vi "path steer51.vi"(11 "lane":bool) -> (2 "curve vel limit":dbl=14.843332236967187, 3 "handle":dbl=-359.09688121459806)   [LabVIEW 2015]
uses:
  G_ALL.vi
  <vilib>/Analysis/polynomials.llb/1D Polynomial Evaluation (DBL).vi
  <vilib>/Analysis/polynomials.llb/nth Derivative of Polynomial (DBL).vi
  <vilib>/Analysis/polynomials.llb/Scalar Polynomial Evaluation (DBL).vi
  G_LCM.vi
  <vilib>/Analysis/NI_AALPro.lvlib
panel:
  in  "index (row)":i32
  out "Array 2":i32[](array[numeric])
  out "Polynomial Coefficients 3":dbl[][](array[numeric])
  out "Array":dbl[](array[numeric])
  out "dist speed":dbl[](array[numeric])=[-6.280629727990325, -5.767652620171672, -5.260811269352596, -4.750405616087261, -4.247626177640517, -3.7442417201726186, -3.234236998487254, -2.733202494381619, -2.2309876435732536, -1.727969770767316, -1.2170174151123292, -0.7112755506690004, -0.2048354308747279, 0.2980698513495696, 0.8052753145152414, 1.3068201262418702, 1.8071308154794987, 2.3105942059932456, 2.816881132611934, 3.321235349091914, 3.8262467144530254, 4.328309326210711, 4.83288013729348, 5.334580351902129, 5.8405154661100145, 6.344513436357381, 6.84671687285963, 7.347037647467956, 7.85260944831298, 8.355677730085302, 8.85924459600933, 9.36378646133383, 9.871392236798886, 10.379135157785838, 10.885149114578343, 11.386372469681485, 11.889282638845971, 12.390546046536894, 12.8945305329367, 13.394897794033318, 13.897303578434707, 14.398578387722258, 14.903133677335356, 15.408547950712162, 15.909840311837332, 16.412650077140604, 16.91886527417174, 17.42043178538479, 17.928892627599016, 18.429060187867897, 18.938769393907265, 19.44497971039645, 19.95108288625684, 20.458874628420645, 20.966711680341415, 21.468694651165553, 21.97077515459592, 22.476640025076534, 22.986901398368484, 23.490789085466282, 23.998423060461953, 24.50111144191703, 25.010444092843613]
  out "Polynomial Coefficients 2":dbl[](array[numeric])
  out "R0":dbl
  out "handle 2":dbl=-359.09688121459806
  out "dist":dbl[](array[numeric])=[-6.280629727990325, -5.767652620171672, -5.260811269352596, -4.750405616087261, -4.247626177640517, -3.7442417201726186, -3.234236998487254, -2.733202494381619, -2.2309876435732536, -1.727969770767316, -1.2170174151123292, -0.7112755506690004, -0.2048354308747279, 0.2980698513495696, 0.8052753145152414, 1.3068201262418702, 1.8071308154794987, 2.3105942059932456, 2.816881132611934, 3.321235349091914, 3.8262467144530254, 4.328309326210711, 4.83288013729348, 5.334580351902129, 5.8405154661100145, 6.344513436357381, 6.84671687285963, 7.347037647467956, 7.85260944831298, 8.355677730085302, 8.85924459600933, 9.36378646133383, 9.871392236798886, 10.379135157785838, 10.885149114578343, 11.386372469681485, 11.889282638845971, 12.390546046536894, 12.8945305329367, 13.394897794033318, 13.897303578434707, 14.398578387722258, 14.903133677335356, 15.408547950712162, 15.909840311837332, 16.412650077140604, 16.91886527417174, 17.42043178538479, 17.928892627599016, 18.429060187867897, 18.938769393907265, 19.44497971039645, 19.95108288625684, 20.458874628420645, 20.966711680341415, 21.468694651165553, 21.97077515459592, 22.476640025076534, 22.986901398368484, 23.490789085466282, 23.998423060461953, 24.50111144191703, 25.010444092843613]
  in  "ap[g]":dbl=0.01 format="%#_13g"
  in  "mu":dbl=0.005 format="%#_13g"
  in  "an[g]":dbl=-0.05 format="%#_13g"
  out "Waveform Graph 2":dynamicdata(graph)=[{"t0"=timestamp(3558070004.848593 s since 1904-01-01), "dt"=1.0, "Y"=[2.6999392249698047, 1.6951051020445074, 1.0707905056587288, 0.8180527212240709, 0.9190152508675626, 1.2963877361766827, 1.970624056488019, 3.4965104940836413, 201.6, 201.6, 201.6, 201.6, 201.6, 201.6, 201.6, 201.6, 201.6, 201.6, 201.6, 201.6, 201.6, 201.6, 201.6, 201.6, 201.6, 9.532169956190149, 6.2694973959061215, 4.816384979354145, 3.8625477434998605, 3.1463412301935363, 2.568397389060611, 2.09391085834571, 1.7118919309961866, 1.427834339946269, 1.2511128718613436, 1.190295122332855, 1.2494808598163556, 1.4335700986818793, 1.7728772048959551, 2.418642872855935, 5.241778140587992, 201.6, 201.6, 201.6, 201.6, 201.6, 201.6, 201.6, 201.6, 201.6, 201.6, 201.6, 201.6, 201.6, 201.6, 201.6, 201.6, 201.6, 201.6, 201.6, 201.6, 201.6, 201.6]}, {"t0"=timestamp(3558070004.848593 s since 1904-01-01), "dt"=1.0, "Y"=[2.6999392249698047, 1.6951051020445074, 1.0707905056587288, 0.8180527212240709, 0.9190152508675626, 1.2963877361766827, 1.970624056488019, 3.4965104940836413, 20.777549661712815, 20.247536270100138, 19.694565186792815, 19.13150029565853, 18.550539773696645, 17.955042408424784, 17.333744168195455, 16.696661871332914, 16.035950098109442, 15.342378965317303, 14.611756797060403, 13.845642849689991, 13.03348797188081, 12.172479477913956, 11.240920032490967, 10.230903985827208, 9.099530123436892, 7.81122506851608, 6.2694973959061215, 4.816384979354145, 3.8625477434998605, 3.1463412301935363, 2.568397389060611, 2.09391085834571, 1.7118919309961866, 1.427834339946269, 1.2511128718613436, 1.190295122332855, 1.2494808598163556, 1.4335700986818793, 1.7728772048959551, 2.418642872855935, 5.241778140587992, 201.6, 201.6, 201.6, 201.6, 201.6, 201.6, 201.6, 201.6, 201.6, 201.6, 201.6, 201.6, 201.6, 201.6, 201.6, 201.6, 201.6, 201.6, 201.6, 201.6, 201.6, 201.6]}, {"t0"=timestamp(0 s since 1904-01-01), "dt"=1.0, "Y"=[2.6999392249698047, 1.6951051020445074, 1.0707905056587288, 0.8180527212240709, 0.9190152508675626, 1.2963877361766827, 1.970624056488019, 3.4965104940836413, 7.108855050211476, 9.429067355168725, 11.308583683012714, 12.902067626338482, 14.32116957022803, 15.603166352532973, 16.797313219711075, 16.696661871332914, 16.035950098109442, 15.342378965317303, 14.611756797060403, 13.845642849689991, 13.03348797188081, 12.172479477913956, 11.240920032490967, 10.230903985827208, 9.099530123436892, 7.81122506851608, 6.2694973959061215, 4.816384979354145, 3.8625477434998605, 3.1463412301935363, 2.568397389060611, 2.09391085834571, 1.7118919309961866, 1.427834339946269, 1.2511128718613436, 1.190295122332855, 1.2494808598163556, 1.4335700986818793, 1.7728772048959551, 2.418642872855935, 5.241778140587992, 8.106464321213798, 10.208013173205686, 11.948130714804863, 13.453538277833673, 14.81058095698709, 16.061404030280418, 17.21131827924602, 18.303446987203408, 19.317614592377343, 20.299067875936583, 21.228923087902636, 22.11953935666036, 22.978461118838254, 23.806486212234905, 24.597587927766437, 25.364173907146245, 26.113789179785613, 26.848724907341754, 27.555251257689754, 28.249167970580274, 28.919921293974994, 29.58403363562809]}]
  out "map_track for speed":dbl[][](array[numeric])=[[-0.3545450857664302, -6.2388566107065655], [-0.27704582904833586, -5.731767488012998], [-0.20533240909466363, -5.230025183339917], [-0.13399376942622507, -4.724629566643976], [-0.06871872109144915, -4.226105412976658], [-0.005201324439524461, -3.7267443688985153], [0.05648658324735591, -3.2204841411632317], [0.11292137912439827, -2.7226380925511173], [0.1614318645585973, -2.2227716212056117], [0.20611921619876952, -1.7217426590032276], [0.2514800464586248, -1.2128077861289897], [0.2966935930855752, -0.7090910317401496], [0.3370616547081277, -0.204262333528494], [0.37465481783960886, 0.29723589874642653], [0.4044573002719885, 0.803565034690598], [0.43241637259429494, 1.3043299380582118], [0.4571121863051213, 1.8040307510959646], [0.45201550718714745, 2.307468343503967], [0.3863546760099802, 2.809479406443939], [0.25417130196906557, 3.2962038986449116], [0.06111432793630125, 3.7628573931364953], [-0.19013433422201217, 4.19753080604394], [-0.49758286654376527, 4.597614676463535], [-0.8530000954510649, 4.951707459126808], [-1.2554532803579177, 5.2583045461104865], [-1.6928943683564668, 5.508622840575976], [-2.155745510638023, 5.703500011438359], [-2.634513106918592, 5.848766890858279], [-3.129308121801891, 5.952597228699951], [-3.627772088541141, 6.020504297462557], [-4.130029041586696, 6.056802252968919], [-4.634539834160694, 6.06240172093335], [-5.142102959732917, 6.055821687131267], [-5.649843095559644, 6.057503437117642], [-6.155823778443234, 6.063306282752706], [-6.656719729677723, 6.081419751160103], [-7.158588084773581, 6.113773922489787], [-7.651740703683538, 6.203582042123632], [-8.131423336348554, 6.35819424879321], [-8.583409716824091, 6.572846776944994], [-9.005194999840848, 6.845809681440183], [-9.386776083797882, 7.170882459126112], [-9.72476913428849, 7.54549791275371], [-10.011412061388244, 7.961766359884512], [-10.239416063440592, 8.40820583660063], [-10.40783468222519, 8.881970365592638], [-10.516838106738941, 9.376310409640807], [-10.590206702194822, 9.872481765496081], [-10.62912705284488, 10.379450831978916], [-10.637432741269066, 10.879549426143232], [-10.61938203200132, 11.388938910345853], [-10.592347246602534, 11.894426798329851], [-10.558291863385081, 12.399382890965526], [-10.517428444424214, 12.90552776587841], [-10.478548864380736, 13.41187433647924], [-10.440437467355913, 13.912408475588894], [-10.405933723810719, 14.413302000807835], [-10.372241554466061, 14.918043622740504], [-10.343427469450347, 15.427490791324738], [-10.315674147163909, 15.930613593740642], [-10.290940898551378, 16.43764467659748], [-10.26753174415437, 16.939787704369788], [-10.243318891221465, 17.44854450978152]]
  out "Polynomial Coefficients":dbl[](array[numeric])=[0.3514314245197786, 0.08317550338697662, -0.0038021171840465, -0.00346461088477799, -0.0012982677212205788, -0.00011561582792426496]
  out "XY Graph":cluster{"Y":dbl[], "Y":dbl[]}[](graph)=[{"Y"=[-0.3545450857664302, -0.27704582904833586, -0.20533240909466363, -0.13399376942622507, -0.06871872109144915, -0.005201324439524461, 0.05648658324735591, 0.11292137912439827, 0.1614318645585973, 0.20611921619876952, 0.2514800464586248, 0.2966935930855752, 0.3370616547081277, 0.37465481783960886, 0.4044573002719885, 0.43241637259429494, 0.4571121863051213, 0.45201550718714745, 0.3863546760099802, 0.25417130196906557, 0.06111432793630125, -0.19013433422201217, -0.49758286654376527, -0.8530000954510649, -1.2554532803579177, -1.6928943683564668], "Y"=[-6.2388566107065655, -5.731767488012998, -5.230025183339917, -4.724629566643976, -4.226105412976658, -3.7267443688985153, -3.2204841411632317, -2.7226380925511173, -2.2227716212056117, -1.7217426590032276, -1.2128077861289897, -0.7090910317401496, -0.204262333528494, 0.29723589874642653, 0.803565034690598, 1.3043299380582118, 1.8040307510959646, 2.307468343503967, 2.809479406443939, 3.2962038986449116, 3.7628573931364953, 4.19753080604394, 4.597614676463535, 4.951707459126808, 5.2583045461104865, 5.508622840575976]}, {"Y"=[-0.34824861454222367, -0.2838190821086385, -0.21088307053199773, -0.13573975147394757, -0.06474548918773154, 0.0006618412479036939, 0.06025418227747581, 0.11267247761975072, 0.16039640436065217, 0.20497730506502992, 0.2486380781866307, 0.29146844512109193, 0.33431047405158726, 0.3757168715400785, 0.41343550897313974, 0.4415691081325965, 0.4528064519658091, 0.43617827243140883, 0.3771483424612058, 0.2619623140505302, 0.07848992524601944, -0.17634937336605716, -0.5008339909423127, -0.875287479505389, -1.27737354646982, -1.6668168609056053], "Y"=[-6.2388566107065655, -5.731767488012998, -5.230025183339917, -4.724629566643976, -4.226105412976658, -3.7267443688985153, -3.2204841411632317, -2.7226380925511173, -2.2227716212056117, -1.7217426590032276, -1.2128077861289897, -0.7090910317401496, -0.204262333528494, 0.29723589874642653, 0.803565034690598, 1.3043299380582118, 1.8040307510959646, 2.307468343503967, 2.809479406443939, 3.2962038986449116, 3.7628573931364953, 4.19753080604394, 4.597614676463535, 4.951707459126808, 5.2583045461104865, 5.508622840575976]}]
  out "ref":dbl[](array[numeric])=[-29.50710129286377, 0.08298448837840622, 0.3514314245197786]
  in  "gain":dbl[](array[numeric])=[0.7, 1400.0, 750.0]
  out "path end":bool
  out "map_track for steering":dbl[][](array[numeric])=[[-0.3545450857664302, -6.2388566107065655], [-0.27704582904833586, -5.731767488012998], [-0.20533240909466363, -5.230025183339917], [-0.13399376942622507, -4.724629566643976], [-0.06871872109144915, -4.226105412976658], [-0.005201324439524461, -3.7267443688985153], [0.05648658324735591, -3.2204841411632317], [0.11292137912439827, -2.7226380925511173], [0.1614318645585973, -2.2227716212056117], [0.20611921619876952, -1.7217426590032276], [0.2514800464586248, -1.2128077861289897], [0.2966935930855752, -0.7090910317401496], [0.3370616547081277, -0.204262333528494], [0.37465481783960886, 0.29723589874642653], [0.4044573002719885, 0.803565034690598], [0.43241637259429494, 1.3043299380582118], [0.4571121863051213, 1.8040307510959646], [0.45201550718714745, 2.307468343503967], [0.3863546760099802, 2.809479406443939], [0.25417130196906557, 3.2962038986449116], [0.06111432793630125, 3.7628573931364953], [-0.19013433422201217, 4.19753080604394], [-0.49758286654376527, 4.597614676463535], [-0.8530000954510649, 4.951707459126808], [-1.2554532803579177, 5.2583045461104865], [-1.6928943683564668, 5.508622840575976]]
  in  "control point":dbl=0.3 format="%#_13g"
  out "R_new":dbl=-132.87270287440214
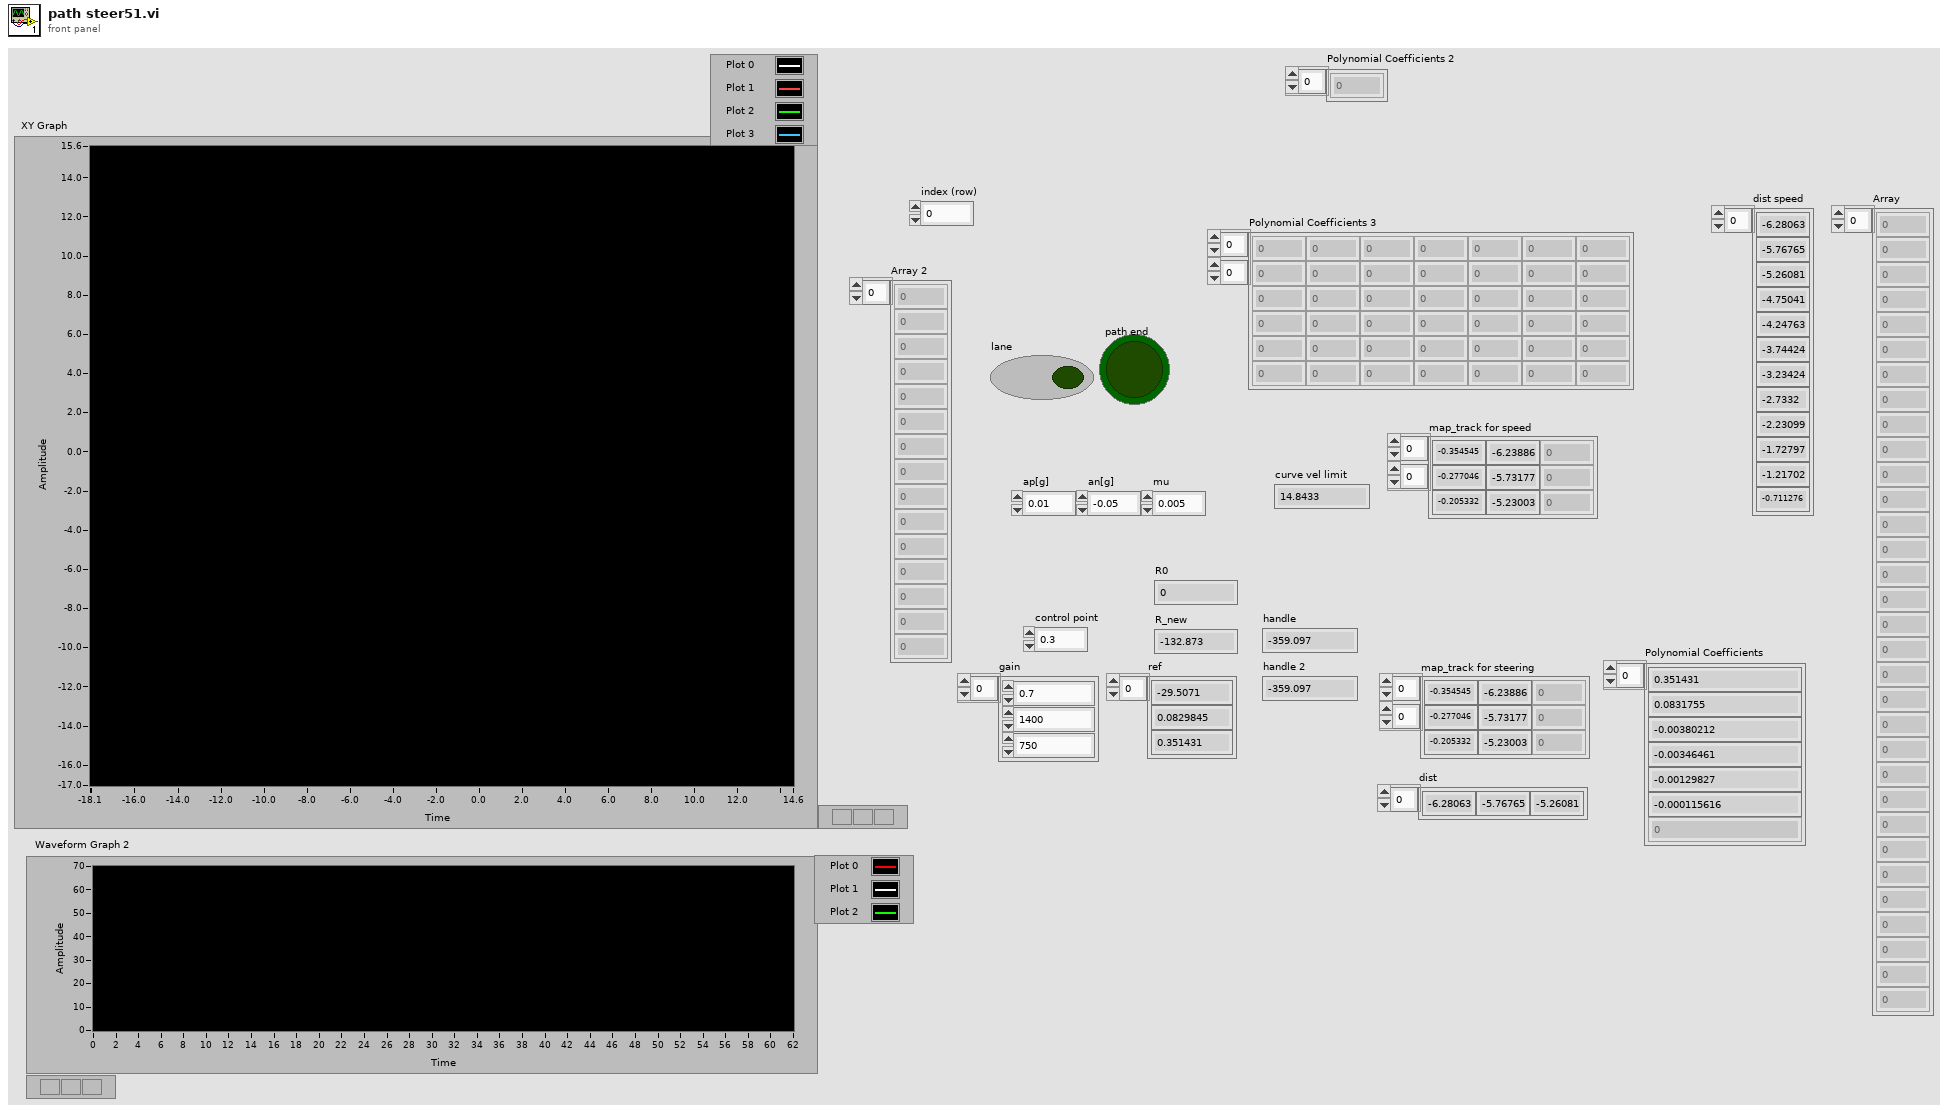
[diagram p1: front panel]
types:
  T1 = cluster{"Steer_input":dbl, "Steer_output":dbl, "VS_des":dbl, "VS_can":dbl, "heading":dbl, "auto":bool, "run":bool, "x":dbl, "y":dbl, "slam_y":dbl, "slam_x":dbl, "slam_heading":dbl}
  T2 = cluster{"C_Wheel base":dbl, "ratio_steer":dbl, "Overall width":dbl, "af":dbl, "turn radius":dbl, "eval":dbl, "ap":dbl, "an":dbl, "Vmax":dbl, "mu":dbl, "Vlast":dbl}
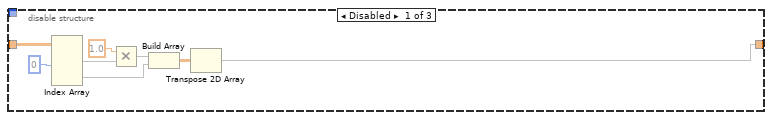
[diagram p2: hidden frame]
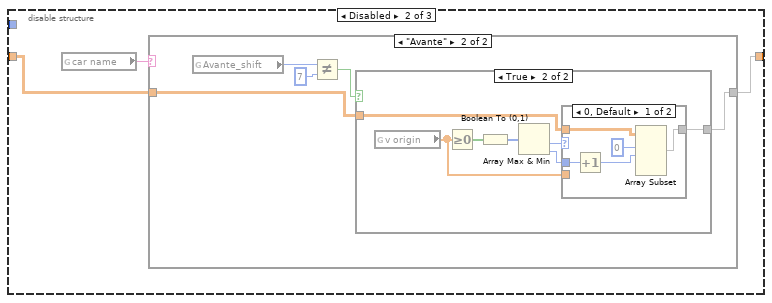
[diagram p3: hidden frame]
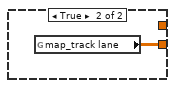
[diagram p7: hidden frame]
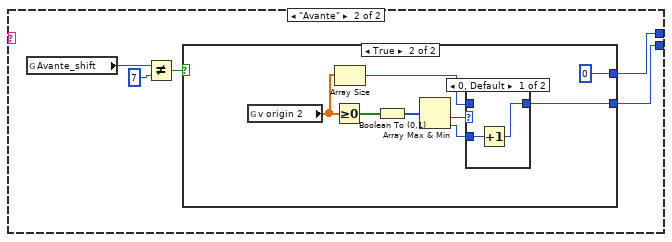
[diagram p9: hidden frame]
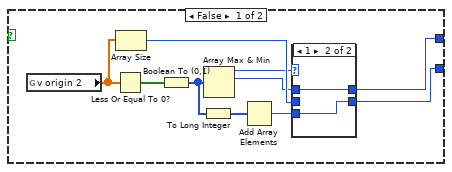
[diagram p10: hidden frame]
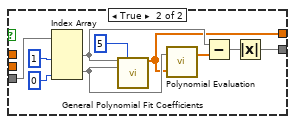
[diagram p14: hidden frame]
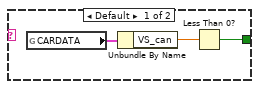
[diagram p17: hidden frame]
diagram:
  n1 = flat-sequence {
    tunnel: [w193] -> w1
    tunnel: w1 -> [w282]
    tunnel: [w357] -> w5
    tunnel: w5 -> [w373]
    tunnel: [w373] -> w4
    tunnel: [w364] -> w3
    tunnel: [w368] -> w2
    tunnel: w4 -> [w405]
    tunnel: w3 -> [w403]
    tunnel: w2 -> [w391]
    frame #0 {
      n2 = case shown="False" "lane" {
        tunnel: [w73 w116] -> w30
        tunnel: [w75 _] -> w64
        frame False {
          n3 = global read "G_ALL.vi" "current idx"() -> (w76:i32)
          n4 = Subtract(x=w76, y=2) -> (x-y=w83:i32)
          n5 = global read "G_ALL.vi" "map_track"() -> (w74:dbl[][])
          n6 = Max & Min(x=w83, y=0) -> (max(x,y)=w71:i32)  [unwired: 1 out]
          n7 = disable-structure shown="Enabled" {
            disable-tunnel: w74 -> [w92 w94 w115]
            disable-tunnel: [w85 w93 w115] -> w73
            disable-tunnel: w71 -> [_ _ _]
            frame Disabled {
              n8 = Index Array(array=w92, index (col) #1=0 ("disabled index (col)")) -> (element #1=w90:dbl[], element #2=w87:dbl[])  [unwired: 3 in]
              n9 = Multiply(x=1.0, y=w90) -> (x*y=w88:dbl[])
              n10 = Build Array(w88, w87) -> (w86:dbl[][])
              n11 = Transpose 2D Array(2D array=w86) -> (transposed array=w85:dbl[][])
            }
            frame Disabled {
              n12 = global read "G_LCM.vi" "car name"() -> (w95:string)
              n13 = case shown="\"Avante\"" w95 {
                tunnel: [w96 w98] -> w93
                tunnel: w94 -> [w96 w97]
                frame Default {
                }
                frame "Avante" {
                  n14 = global read "G_ALL.vi" "Avante_shift"() -> (w100:u8)
                  n15 = Not Equal?(x=w100, y=u8 7) -> (x != y?=w99:bool)
                  n16 = case shown="True" w99 {
                    tunnel: [_ w104] -> w98
                    tunnel: w97 -> [_ w103]
                    frame False {
                    }
                    frame True {
                      n17 = global read "G_ALL.vi" "v origin"() -> (w105:dbl[])
                      n18 = Greater Or Equal To 0?(x=w105) -> (x >= 0?=w108:bool[])
                      n19 = Boolean To (0,1)(Boolean=w108) -> (0, 1=w107:i16[])
                      n20 = Array Max & Min(array=w107) -> (min value=w106:i16, min index (indices)=w102:i32)  [unwired: 2 out]
                      n21 = case shown="0, Default" w106 {
                        tunnel: w105 -> [_ _]
                        tunnel: [w110 w114] -> w104
                        tunnel: w103 -> [w112 w114]
                        tunnel: w102 -> [w113 _]
                        frame 0, Default {
                          n22 = Increment(x=w113) -> (x+1=w111:i32)
                          n23 = Array Subset(array=w112, index (row)=0 ("index"), length (row)=w111) -> (w110:dbl[][])  [unwired: 2 in]
                        }
                        frame 1 {
                        }
                      }
                    }
                  }
                }
              }
            }
            frame Enabled {
            }
          }
          n24 = Array Subset(array=w73, index (row)=w71, length (row)=5 ("length")) -> (w80:dbl[][])  [unwired: 2 in]
          n25 = Index Array(array=w80, index (col)=1 ("disabled index (col)")) -> (element=w78:dbl[])  [unwired: 1 in]
          n26 = Threshold 1D Array(2:0.0 ("threshold y"), 3:w78) -> (0:w72:dbl)  [unwired: 1 in]
          n27 = Add(x=w71, y=w72) -> (x+y=w75:dbl)
        }
        frame True {
          n28 = global read "G_ALL.vi" "map_track lane"() -> (w116:dbl[][])
        }
      }
      n29 = Round Toward -Infinity(1:w64) -> (0:w59:dbl)
      n30 = Index Array(array=w30, index (col) #1=0 ("disabled index (col)")) -> (element #1=w22:dbl[], element #2=w23:dbl[])  [unwired: 3 in]
      n31 = Equal?(x=w59, y=w64) -> (x = y?=w60:bool)
      n32 = To Long Integer(number=w59) -> (32bit integer=w61:i32)
      n33 = Interpolate 1D Array(1:w64, 2:w22) -> (0:w24:dbl)
      n34 = Interpolate 1D Array(1:w64, 2:w23) -> (0:w25:dbl)
      n35 = Increment(x=w61) -> (x+1=w62:i32)
      n36 = Round Toward +Infinity(x=w64) -> (ceil(x): smallest int >= x=w58:dbl)
      n37 = Select(t=w61, s=w60, f=w62) -> (s? t:f=w18:i32)
      n38 = global read "G_ALL.vi" "CARDATA"() -> (w28:T1)
      n39 = Array Subset(array=w30, index (row)=0 ("index"), length (row)=w18) -> (w32:dbl[][])  [unwired: 2 in]
      n40 = Unbundle By Name(w28) -> ("VS_can"=w65:dbl)
      n41 = Index Array(array=w32, index (col) #1=0 ("disabled index (col)")) -> (element #1=w34:dbl[], element #2=w35:dbl[])  [unwired: 3 in]
      n42 = Reverse 1D Array(array=w34) -> (reversed array=w36:dbl[])
      n43 = Reverse 1D Array(array=w35) -> (reversed array=w37:dbl[])
      n44 = Multiply(x=2.0, y=w65) -> (x*y=w66:dbl)
      n45 = Build Array(w36, w37) -> (w56:dbl[][])
      n46 = To Long Integer(number=w58) -> (32bit integer=w9:i32)
      n47 = Max & Min(x=w66, y=25.0) -> (max(x,y)=w29:dbl)  [unwired: 1 out]
      n48 = Array Subset(array=w30, index (row)=w9) -> (w54:dbl[][])  [unwired: 3 in]
      n49 = Transpose 2D Array(2D array=w56) -> (transposed array=w57:dbl[][])
      n50 = Build Array(w24, w25) -> (w39:dbl[])
      n51 = for {
        tunnel: w57 -> [w119] mode=indexing
        shift-right: [w119] -> _
        shift-left: w39 -> [w126]
        shift-right: [w118] -> _
        shift-left: 0.0 -> [w121]
        tunnel: 15.0 ("y") -> [w120]
        tunnel: [w118] -> w43 mode=indexing
        stop <- w117 stop-if-true
        n52 = Subtract(x=w119, y=w126) -> (x-y=w125:dbl[])
        n53 = Square(x=w125) -> (x^2=w124:dbl[])
        n54 = Add Array Elements(numeric array=w124) -> (sum=w123:dbl)
        n55 = Square Root(x=w123) -> (sqrt(x)=w122:dbl)
        n56 = Add(x=w121, y=w122) -> (x+y=w118:dbl)
        n57 = Greater Or Equal?(x=w118, y=w120) -> (x >= y?=w117:bool)
      }
      n58 = for {
        tunnel: w54 -> [w129] mode=indexing
        shift-right: [w129] -> _
        shift-left: w39 -> [w136]
        shift-right: [w128] -> _
        shift-left: 0.0 -> [w131]
        tunnel: w29 -> [w130]
        tunnel: [w128] -> w55 mode=indexing
        tunnel: [w127] -> w69
        stop <- w127 stop-if-true
        n59 = Subtract(x=w129, y=w136) -> (x-y=w135:dbl[])
        n60 = Square(x=w135) -> (x^2=w134:dbl[])
        n61 = Add Array Elements(numeric array=w134) -> (sum=w133:dbl)
        n62 = Square Root(x=w133) -> (sqrt(x)=w132:dbl)
        n63 = Add(x=w131, y=w132) -> (x+y=w128:dbl)
        n64 = Greater Or Equal?(x=w128, y=w130) -> (x >= y?=w127:bool)
      }
      n65 = global read "G_ALL.vi" "v origin"() -> (w10:dbl[])
      n66 = Array Subset(array=w10, index=0, length=w18) -> (w16:dbl[])
      n67 = Negate(x=w43) -> (-x=w41:dbl[])
      n68 = Not(x=w69) -> (.not. x?=→"path end":bool)
      n69 = Array Size(array=w43) -> (size(s)=w13:i32)
      n70 = Array Size(array=w55) -> (size(s)=w8:i32)
      n71 = Reverse 1D Array(array=w16) -> (reversed array=w15:dbl[])
      n72 = Array Subset(array=w10, index=w9, length=w8) -> (w7:dbl[])
      n73 = Reverse 1D Array(array=w41) -> (reversed array=w42:dbl[])
      n74 = Array Subset(array=w57, index (row)=0 ("index"), length (row)=w13) -> (w49:dbl[][])  [unwired: 2 in]
      n75 = Array Subset(array=w54, index (row)=0 ("index"), length (row)=w8) -> (w68:dbl[][])  [unwired: 2 in]
      n76 = Build Array (concatenate)(w42, w55) -> (w19:dbl[])
      n77 = Array Subset(array=w15, index=0, length=w13) -> (w12:dbl[])
      n78 = global write "G_ALL.vi" "dist"(w19) -> ()
      n79 = Reverse 1D Array(array=w12) -> (reversed array=w11:dbl[])
      n80 = Index Array(array=w49, index (col) #1=0 ("disabled index (col)")) -> (element #1=w50:dbl[], element #2=w51:dbl[])  [unwired: 3 in]
      n81 = Reverse 1D Array(array=w50) -> (reversed array=w47:dbl[])
      n82 = Reverse 1D Array(array=w51) -> (reversed array=w46:dbl[])
      n83 = Build Array (concatenate)(w11, w7) -> (w6:dbl[])
      n84 = Build Array(w47, w46) -> (w45:dbl[][])
      n85 = global write "G_ALL.vi" "v origin 2"(w6) -> ()
      n86 = Transpose 2D Array(2D array=w45) -> (transposed array=w52:dbl[][])
      n87 = Build Array (concatenate)(w52, w68) -> (w20:dbl[][])
      n88 = global write "G_ALL.vi" "map_track 2"(w20) -> ()
    }
    frame #1 {
      n89 = disable-structure shown="Disabled" {
        disable-tunnel: [w157 _] -> w145
        frame Disabled {
          n90 = global read "G_LCM.vi" "car name"() -> (w157:string)
        }
        frame Enabled {
        }
      }
      n91 = case shown="\"False\", Default" w145 {
        tunnel: [w158 w162] -> w141
        tunnel: [_ w161] -> w140
        frame "False", Default {
          n92 = global read "G_ALL.vi" "dist"() -> (w159:dbl[])
          n93 = Array Size(array=w159) -> (size(s)=w158:i32)
        }
        frame "Avante" {
          n94 = global read "G_ALL.vi" "Avante_shift"() -> (w163:u8)
          n95 = Not Equal?(x=w163, y=u8 7) -> (x != y?=w160:bool)
          n96 = case shown="True" w160 {
            tunnel: [w168 w183] -> w162
            tunnel: [w172 0] -> w161
            frame False {
              n97 = global read "G_ALL.vi" "v origin 2"() -> (w174:dbl[])
              n98 = Less Or Equal To 0?(x=w174) -> (x <= 0?=w169:bool[])
              n99 = Array Size(array=w174) -> (size(s)=w173:i32)
              n100 = Boolean To (0,1)(Boolean=w169) -> (0, 1=w166:i16[])
              n101 = To Long Integer(number=w166) -> (32bit integer=w165:i32[])
              n102 = Array Max & Min(array=w166) -> (max value=w170:i16, max index (indices)=w171:i32)  [unwired: 2 out]
              n103 = Add Array Elements(numeric array=w165) -> (sum=w167:i32)
              n104 = case shown="1" w170 {
                tunnel: w173 -> [w175 _]
                tunnel: [_ w177] -> w172
                tunnel: w171 -> [_ w177]
                tunnel: [w175 w176] -> w168
                tunnel: w167 -> [_ w176]
                frame 0, Default {
                }
                frame 1 {
                }
              }
            }
            frame True {
              n105 = global read "G_ALL.vi" "v origin 2"() -> (w180:dbl[])
              n106 = Greater Or Equal To 0?(x=w180) -> (x >= 0?=w185:bool[])
              n107 = Array Size(array=w180) -> (size(s)=w184:i32)
              n108 = Boolean To (0,1)(Boolean=w185) -> (0, 1=w182:i16[])
              n109 = Array Max & Min(array=w182) -> (min value=w181:i16, min index (indices)=w178:i32)  [unwired: 2 out]
              n110 = case shown="0, Default" w181 {
                tunnel: w184 -> [_ w188]
                tunnel: [w187 w188] -> w183
                tunnel: w178 -> [w186 _]
                frame 0, Default {
                  n111 = Increment(x=w186) -> (x+1=w187:i32)
                }
                frame 1 {
                }
              }
            }
          }
        }
      }
      n112 = global read "G_ALL.vi" "dist"() -> (w144:dbl[])
      n113 = Array Subset(array=w144, index=w140, length=w141) -> (w137:dbl[])
      "dist speed" <- w137
      n114 = Threshold 1D Array(2:-6.0 ("threshold y"), 3:w137) -> (0:w155:dbl)  [unwired: 1 in]
      n115 = Round Toward -Infinity(1:w155) -> (0:w156:dbl)
      n116 = To Long Integer(number=w156) -> (32bit integer=w147:i32)
      n117 = Array Subset(array=w137, index=w147) -> (→"dist":dbl[])  [unwired: 1 in]
      n118 = Threshold 1D Array(1:w147, 2:6.0 ("threshold y"), 3:w137) -> (0:w150:dbl)
      n119 = Round Toward +Infinity(x=w150) -> (ceil(x): smallest int >= x=w149:dbl)
      n120 = global read "G_ALL.vi" "map_track 2"() -> (w143:dbl[][])
      n121 = To Long Integer(number=w149) -> (32bit integer=w151:i32)
      n122 = Subtract(x=w151, y=w147) -> (x-y=w152:i32)
      n123 = Increment(x=w152) -> (x+1=w153:i32)
      n124 = Array Subset(array=w143, index (row)=w140) -> (w142:dbl[][])  [unwired: 3 in]
      n125 = Array Subset(array=w142, index (row)=w147) -> (→"map_track for speed":dbl[][])  [unwired: 3 in]
      n126 = Array Subset(array=w142, index (row)=w147, length (row)=w153) -> (→"map_track for steering":dbl[][])  [unwired: 2 in]
    }
    frame #2 {
      n127 = local read "dist speed"() -> (w198:dbl[])
      n128 = local read "map_track for speed"() -> (w199:dbl[][])
      n129 = Multiply(x=w198, y=0.0) -> (x*y=w196:dbl[])
      n130 = Add(x=w196, y=inf) -> (x+y=w194:dbl[])
      n131 = while {
        shift-right: [w210] -> _
        shift-left: w199 -> [w217]
        tunnel: w198 -> [w214]
        shift-right: [w211] -> w193
        shift-left: w194 -> [w213]
        tunnel: [w212] -> w192 mode=indexing
        tunnel: [w200] -> w189 mode=indexing
        stop <- w204 stop-if-true
        n132 = Array Size(array=w217) -> (size(s)=w219:i32[])
        n133 = Index Array(array=w219, index=0) -> (element=w215:i32)
        n134 = while {
          tunnel: w217 -> [w254]
          shift-right: [w252] -> _
          shift-left: w215 -> [w248]
          tunnel: [w248] -> w200
          tunnel: [w241] -> w212
          stop <- w250 stop-if-true
          n135 = disable-structure shown="Enabled" {
            disable-tunnel: w254 -> [w275 w277]
            disable-tunnel: [w274 w277] -> w247
            disable-tunnel: w248 -> [w273 _]
            frame Enabled {
              n136 = Array Subset(array=w275, index (row)=0 ("index"), length (row)=w273) -> (w274:dbl[][])  [unwired: 2 in]
            }
            frame Disabled {
            }
          }
          n137 = Scale By Power Of 2(n=i16 -1, x=w248) -> (x*2^n=w252:i32)
          n138 = Index Array(array=w247, index (col) #1=0 ("disabled index (col)")) -> (element #1=w258:dbl[], element #2=w256:dbl[])  [unwired: 3 in]
          n139 = call <vilib>:"General Polynomial Fit Coefficients.vi"("Y"=w258, "polynomial order"=5, "X"=w256) -> ("Polynomial Coefficients"=w240:dbl[])  [unwired: 11 in, 1 out]
          n140 = call-poly <vilib>:"Polynomial Evaluation.vi"("P(x)"=w240, "A"=w256) -> ("P(A)"=w255:dbl[])  [unwired: 1 out]
          n141 = Index Array(array=w240, index=5) -> (element=w239:dbl)
          n142 = Absolute Value(x=w239) -> (abs(x)=w238:dbl)
          n143 = Subtract(x=w258, y=w255) -> (x-y=w257:dbl[])
          n144 = Absolute Value(x=w257) -> (abs(x)=w242:dbl[])
          n145 = Greater Or Equal?(x=w238, y=1.0) -> (x >= y?=w244:bool)
          n146 = case shown="False" w244 {
            tunnel: w247 -> [_ w266]
            tunnel: [w262 w264] -> w243
            tunnel: w242 -> [w262 _]
            tunnel: [w261 w263] -> w241
            tunnel: w240 -> [w261 _]
            frame False {
            }
            frame True {
              n147 = Index Array(array=w266, index (col) #1=1 ("disabled index (col)"), index (col) #2=0 ("index (col)")) -> (element #1=w269:dbl[], element #2=w271:dbl[])  [unwired: 2 in]
              n148 = call <vilib>:"General Polynomial Fit Coefficients.vi"("Y"=w269, "polynomial order"=5, "X"=w271) -> ("Polynomial Coefficients"=w263:dbl[])  [unwired: 11 in, 1 out]
              n149 = call-poly <vilib>:"Polynomial Evaluation.vi"("P(x)"=w263, "A"=w271) -> ("P(A)"=w272:dbl[])  [unwired: 1 out]
              n150 = Subtract(x=w269, y=w272) -> (x-y=w270:dbl[])
              n151 = Absolute Value(x=w270) -> (abs(x)=w264:dbl[])
            }
          }
          n152 = Array Max & Min(array=w243) -> (max value=w251:dbl)  [unwired: 3 out]
          n153 = Less?(x=w251, y=0.05) -> (x < y?=w250:bool)
        }
        n154 = Less Or Equal?(x=w200, y=5) -> (x <= y?=w201:bool)
        n155 = Delete From Array(array=w217, length=w200, index (row)=0) -> (array with subset deleted=w210:dbl[][])  [unwired: 1 in, 1 out]
        n156 = Empty Array?(array=w210) -> (empty?=w206:bool)
        n157 = case shown="False" w201 {
          tunnel: w214 -> [w225 _]
          tunnel: w213 -> [w223 w237]
          tunnel: w212 -> [w221 _]
          tunnel: [w220 w237] -> w211
          frame False {
            n158 = call-poly <vilib>:"nth Derivative of Polynomial.vi"("order"=2, "P(x)"=w221) -> ("Nth Derivative of P(x)"=w228:dbl[])  [unwired: 8 in, 1 out]
            n159 = call-poly <vilib>:"nth Derivative of Polynomial.vi"("order"=1, "P(x)"=w221) -> ("Nth Derivative of P(x)"=w230:dbl[])  [unwired: 8 in, 1 out]
            n160 = call-poly <vilib>:"Polynomial Evaluation.vi"("P(x)"=w228, "A"=w225) -> ("P(A)"=w226:dbl[])  [unwired: 1 out]
            n161 = call-poly <vilib>:"Polynomial Evaluation.vi"("P(x)"=w230, "A"=w225) -> ("P(A)"=w234:dbl[])  [unwired: 1 out]
            n162 = Square(x=w234) -> (x^2=w231:dbl[])
            n163 = Increment(x=w231) -> (x+1=w233:dbl[])
            n164 = Square Root(x=w233) -> (sqrt(x)=w232:dbl[])
            n165 = Multiply(x=w232, y=w233) -> (x*y=w229:dbl[])
            n166 = Divide(x=w226, y=w229) -> (x/y=w236:dbl[])
            n167 = Reciprocal(x=w236) -> (1/x=w224:dbl[])
            n168 = Absolute Value(x=w224) -> (abs(x)=w222:dbl[])
            n169 = Max & Min(x=w222, y=w223) -> (min(x,y)=w220:dbl[])  [unwired: 1 out]
          }
          frame True {
          }
        }
        n170 = Array Size(array=w210) -> (size(s)=w209:i32[])
        n171 = Index Array(array=w209, index=0) -> (element=w203:i32)
        n172 = Less Or Equal?(x=w203, y=5) -> (x <= y?=w205:bool)
        n173 = Compound Arithmetic op=OR(w206, w205) -> (w204:bool)
      }
      "Array" <- w193
      "Polynomial Coefficients 3" <- w192
      "Array 2" <- w189
      n174 = Index Array(array=w192, index (row)="index (row)") -> (element=→"Polynomial Coefficients 2":dbl[])  [unwired: 1 in]
    }
    frame #3 {
      n175 = Compound Arithmetic op=MULTIPLY(w282, 9.81 ("value"), "mu") -> (w305:dbl[])
      n176 = Square Root(x=w305) -> (sqrt(x)=w280:dbl[])
      n177 = In Range and Coerce(upper limit=56.0 ("value"), x=w280, lower limit=0.5) -> (coerced(x)=w281:dbl[])  [unwired: 1 out]
      n178 = local read "path end"() -> (w312:bool)
      n179 = call "Convert to Dynamic Data6"("Array"=w281) -> ("Dynamic Data Type"=w287:dynamicdata)  [unwired: 3 in]
      n180 = Reverse 1D Array(array=w281) -> (reversed array=w313:dbl[])
      n181 = case shown="True" w312 {
        tunnel: w313 -> [w333 w337]
        tunnel: [w333 w336] -> w314
        frame False {
        }
        frame True {
          n182 = Replace Array Subset(array=w337, new element=0.0 ("new element/subarray"), index=0) -> (w336:dbl[])
        }
      }
      n183 = local read "dist speed"() -> (w285:dbl[])
      n184 = Array Size(array=w314) -> (size(s)=w310:i32)
      n185 = Reverse 1D Array(array=w285) -> (reversed array=w307:dbl[])
      n186 = Decrement(x=w310) -> (x-1=w309:i32)
      n187 = Negate(x=w307) -> (-x=w308:dbl[])
      n188 = for {
        N: w309 -> [_]
        tunnel: w314 -> [w353] mode=indexing
        tunnel: w308 -> [w354]
        shift-right: [w344] -> w293
        shift-left: w314 -> [w347]
        tunnel: w308 -> [w341] mode=indexing
        tunnel: "an[g]" -> [w338]
        i -> [w355]
        n189 = Square(x=w353) -> (x^2=w352:dbl)
        n190 = Increment(x=w355) -> (x+1=w346:i32)
        n191 = Array Subset(array=w347, index=w346) -> (w348:dbl[])  [unwired: 1 in]
        n192 = Array Subset(array=w354, index=w346) -> (w342:dbl[])  [unwired: 1 in]
        n193 = Subtract(x=w342, y=w341) -> (x-y=w340:dbl[])
        n194 = Compound Arithmetic op=MULTIPLY(w340, 9.81 ("value"), 2.0 ("value"), w338) -> (w350:dbl[])
        n195 = Subtract(x=w352, y=w350) -> (x-y=w349:dbl[])
        n196 = Square Root(x=w349) -> (sqrt(x)=w343:dbl[])
        n197 = Max & Min(x=w348, y=w343) -> (min(x,y)=w345:dbl[])  [unwired: 1 out]
        n198 = Replace Array Subset(array=w347, new element=w345, index=w346) -> (w344:dbl[])
      }
      n199 = Reverse 1D Array(array=w293) -> (reversed array=w290:dbl[])
      n200 = local read "dist speed"() -> (w284:dbl[])
      n201 = Array Size(array=w290) -> (size(s)=w296:i32)
      n202 = call "Convert to Dynamic Data5"("Array"=w290) -> ("Dynamic Data Type"=w286:dynamicdata)  [unwired: 3 in]
      n203 = Decrement(x=w296) -> (x-1=w297:i32)
      n204 = Negate(x=w284) -> (-x=w292:dbl[])
      n205 = for {
        N: w297 -> [_]
        tunnel: w290 -> [w330] mode=indexing
        tunnel: w292 -> [w331]
        shift-right: [w321] -> w289
        shift-left: w290 -> [w324]
        tunnel: w292 -> [w318] mode=indexing
        tunnel: "ap[g]" -> [w315]
        i -> [w332]
        n206 = Square(x=w330) -> (x^2=w329:dbl)
        n207 = Increment(x=w332) -> (x+1=w323:i32)
        n208 = Array Subset(array=w324, index=w323) -> (w325:dbl[])  [unwired: 1 in]
        n209 = Array Subset(array=w331, index=w323) -> (w319:dbl[])  [unwired: 1 in]
        n210 = Subtract(x=w319, y=w318) -> (x-y=w317:dbl[])
        n211 = Compound Arithmetic op=MULTIPLY(w317, 9.81 ("value"), 2.0 ("value"), w315) -> (w327:dbl[])
        n212 = Subtract(x=w329, y=w327) -> (x-y=w326:dbl[])
        n213 = Square Root(x=w326) -> (sqrt(x)=w320:dbl[])
        n214 = Max & Min(x=w325, y=w320) -> (min(x,y)=w322:dbl[])  [unwired: 1 out]
        n215 = Replace Array Subset(array=w324, new element=w322, index=w323) -> (w321:dbl[])
      }
      n216 = local read "dist speed"() -> (w283:dbl[])
      n217 = Threshold 1D Array(2:0.0 ("threshold y"), 3:w283) -> (0:w301:dbl)  [unwired: 1 in]
      n218 = call "Convert to Dynamic Data7"("Array"=w289) -> ("Dynamic Data Type"=w294:dynamicdata)  [unwired: 3 in]
      n219 = Interpolate 1D Array(1:w301, 2:w289) -> (0:w288:dbl)
      n220 = Merge Signals(w287, w286, w294) -> (w299:dynamicdata)
      n221 = Multiply(x=w288, y=3.6) -> (x*y=→"curve vel limit":dbl)
      n222 = Multiply(x=w299, y=3.6) -> (x*y=→"Waveform Graph 2":dynamicdata)
    }
    frame #4 {
      n223 = local read "map_track for steering"() -> (w363:dbl[][])
      n224 = Index Array(array=w363, index (col) #1=0 ("disabled index (col)")) -> (element #1=w360:dbl[], element #2=w361:dbl[])  [unwired: 3 in]
      n225 = call <vilib>:"General Polynomial Fit Coefficients.vi"("Y"=w360, "polynomial order"=5, "X"=w361) -> ("Polynomial Coefficients"=w356:dbl[])  [unwired: 11 in, 1 out]
      "Polynomial Coefficients" <- w356
      n226 = call-poly <vilib>:"Polynomial Evaluation.vi"("P(x)"=w356, "a"=0.0) -> ("P(a)"=w357:dbl)  [unwired: 1 out]
    }
    frame #5 {
      n227 = global read "G_LCM.vi" "car name"() -> (w369:string)
      n228 = case shown="\"Avante\"" w369 {
        tunnel: [w374 w377] -> w368
        frame Default {
          n229 = global read "G_ALL.vi" "CARDATA"() -> (w376:T1)
          n230 = Unbundle By Name(w376) -> ("VS_can"=w375:dbl)
          n231 = Less Than 0?(x=w375) -> (x < 0?=w374:bool)
        }
        frame "Avante" {
          n232 = global read "G_ALL.vi" "Avante_shift"() -> (w379:u8)
          n233 = Equal?(x=w379, y=u8 7) -> (x = y?=w377:bool)
        }
      }
      n234 = local read "Polynomial Coefficients"() -> (w372:dbl[])
      n235 = Negate(x="control point") -> (-x=w367:dbl)
      n236 = Select(t=w367, s=w368, f="control point") -> (s? t:f=w365:dbl)
      n237 = call-poly <vilib>:"nth Derivative of Polynomial.vi"("order"=1, "P(x)"=w372) -> ("Nth Derivative of P(x)"=w370:dbl[])  [unwired: 8 in, 1 out]
      n238 = call-poly <vilib>:"Polynomial Evaluation.vi"("P(x)"=w370, "a"=w365) -> ("P(a)"=w364:dbl)  [unwired: 1 out]
    }
    frame #6 {
      n239 = Square(x=w403) -> (x^2=w432:dbl)
      n240 = global read "G_ALL.vi" "CARDATA"() -> (w402:T1)
      n241 = Increment(x=w432) -> (x+1=w430:dbl)
      n242 = local read "Polynomial Coefficients"() -> (w404:dbl[])
      n243 = local read "Polynomial Coefficients"() -> (w385:dbl[])
      n244 = Unbundle By Name(w402) -> ("VS_can"=w401:dbl)
      n245 = Square Root(x=w430) -> (sqrt(x)=w431:dbl)
      n246 = Multiply(x=w431, y=w430) -> (x*y=w429:dbl)
      n247 = local read "control point"() -> (w382:dbl)
      n248 = Divide(x=w401, y=3.6) -> (x/y=w422:dbl)
      n249 = Absolute Value(x=w422) -> (abs(x)=w425:dbl)
      n250 = call-poly <vilib>:"nth Derivative of Polynomial.vi"("order"=2, "P(x)"=w404) -> ("Nth Derivative of P(x)"=w380:dbl[])  [unwired: 8 in, 1 out]
      n251 = Index Array(array=w385, index=1) -> (element=w383:dbl)
      n252 = call-poly <vilib>:"Polynomial Evaluation.vi"("P(x)"=w380, "a"=w382) -> ("P(a)"=w381:dbl)  [unwired: 1 out]
      n253 = Square(x=w383) -> (x^2=w388:dbl)
      n254 = Inverse Tangent(1:w383) -> (0:w427:dbl)
      n255 = Max & Min(x=w425, y=1.0) -> (max(x,y)=w423:dbl)  [unwired: 1 out]
      n256 = global read "G_ALL.vi" "CARSPEC"() -> (w417:T2)
      n257 = Divide(x=w405, y=w423) -> (x/y=w406:dbl)
      n258 = Divide(x=w429, y=w381) -> (x/y=w409:dbl)
      "R_new" <- w409
      n259 = Increment(x=w388) -> (x+1=w390:dbl)
      n260 = call "headingoperater.vi"("h1"=w427, "h2"=3.141592653589793) -> ("h2-h1"=w428:dbl)  [unwired: 8 in, 1 out]
      n261 = Unbundle By Name(w417) -> ("ratio_steer"=w419:dbl, "C_Wheel base"=w418:dbl)
      n262 = Select(t=w428, s=w391, f=w427) -> (s? t:f=w407:dbl)
      n263 = Square Root(x=w390) -> (sqrt(x)=w389:dbl)
      n264 = Multiply(x=w389, y=w390) -> (x*y=w387:dbl)
      n265 = Divide(x=w418, y=w409) -> (x/y=w411:dbl)
      n266 = Divide(x=w387, y=w381) -> (x/y=→"R0":dbl)
      n267 = Inverse Tangent(1:w411) -> (0:w413:dbl)
      n268 = Multiply(x=180.0 ("y"), y=w413) -> (x*y=w414:dbl)
      n269 = Divide(x=w414, y=3.141592653589793) -> (x/y=w416:dbl)
      n270 = Multiply(x=w419, y=w416) -> (x*y=w410:dbl)
      n271 = Not A Number/Path/Refnum?(number/path/refnum=w410) -> (NaN/Path/Refnum?=w420:bool)
      n272 = Select(t=0.0, s=w420, f=w410) -> (s? t:f=w408:dbl)
      n273 = Build Array(w408, w407, w406) -> (w399:dbl[])
      "ref" <- w399
      n274 = Multiply(x=w399, y="gain") -> (x*y=w392:dbl[])
      n275 = Add Array Elements(numeric array=w392) -> (sum=w398:dbl)
      "handle 2" <- w398
      n276 = Negate(x=w398) -> (-x=w397:dbl)
      n277 = In Range and Coerce(upper limit=479.0, x=w397, lower limit=-479.0) -> (coerced(x)=→"handle":dbl)  [unwired: 1 out]
    }
    frame #7 {
      n278 = local read "map_track for speed"() -> (w447:dbl[][])
      n279 = local read "Polynomial Coefficients 2"() -> (w436:dbl[])
      n280 = Index Array(array=w447, index (col) #1=0 ("disabled index (col)")) -> (element #1=w445:dbl[], element #2=w437:dbl[])  [unwired: 3 in]
      n281 = local read "R0"() -> (w438:dbl)
      n282 = call-poly <vilib>:"Polynomial Evaluation.vi"("P(x)"=w436, "A"=w437) -> ("P(A)"=w441:dbl[])  [unwired: 1 out]
      n283 = call "Convert to Dynamic Data"("Array"=w445) -> ("Dynamic Data Type"=w444:dynamicdata)  [unwired: 3 in]
      n284 = call "Convert to Dynamic Data2"("Array"=w437) -> ("Dynamic Data Type"=w443:dynamicdata)  [unwired: 3 in]
      n285 = call "Convert to Dynamic Data3"("Array"=w437) -> ("Dynamic Data Type"=w442:dynamicdata)  [unwired: 3 in]
      n286 = Merge Signals(w443, w442) -> (w435:dynamicdata)
      n287 = Build Array (concatenate)(w438, w436) -> (w439:dbl[])
      n288 = call "Convert to Dynamic Data4"("Array"=w441) -> ("Dynamic Data Type"=w440:dynamicdata)  [unwired: 3 in]
      n289 = global write "G_ALL.vi" "Steering coeff"(w439) -> ()
      n290 = Merge Signals(w444, w440) -> (w434:dynamicdata)
      n291 = call "Build XY Graph"("Y Input"=w435, "X Input"=w434) -> ("XY Graph"=→"XY Graph":cluster{"X":dbl[], "Y":dbl[]}[])  [unwired: 8 in, 1 out]
    }
  }
